vi "Day 6.2 - .vi"(11 "input":string) -> (3 "output":i16)   [LabVIEW 2021]
uses:
  c0392e8e-aec3-4db0-a7c0-dbb49c44d685.vi
  <vilib>/Comparison/Less/Less Functor/Less Functor.lvclass
panel:
  # "mjqjpqmgbljsphdztnvjfqwrcgsmlb: first marker after character 19\nbvwbjplbgvbhsrlpgdmjqwftvncz: first marker after character 23\nnppdvjthqldpwncqszvftbrmjlhg: first marker after character 23\nnznrnfrfntjfmvfwmzdfjlvtqnbhcprsg: first marker after character 29\nzcfzfwzzqfrljwzlrfnpqdbhtmscgvjw: first marker after character 26"
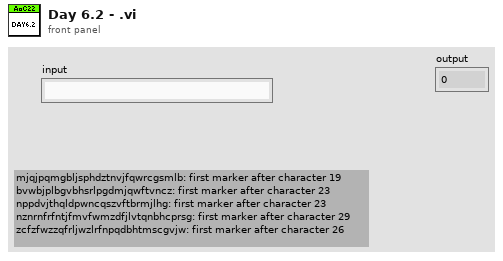
[diagram p1: front panel]
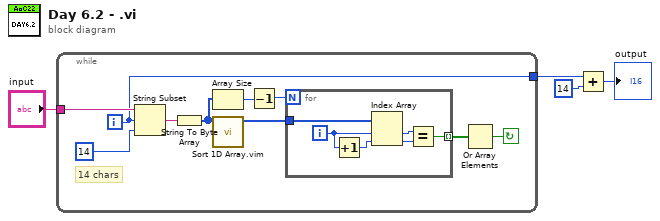
[diagram p0: block diagram]
diagram:
  n1 = while {
    tunnel: "input" -> [w14]
    tunnel: [w11] -> w3
    i -> [w11]
    stop <- w5 continue-if-true
    # "14 chars"
    n2 = String Subset(string=w14, offset (0)=w11, length (rest)=14 ("length (rest)")) -> (substring=w12:string)
    n3 = String To Byte Array(string=w12) -> (unsigned byte array=w9:u8[])
    n4 = Array Size(array=w9) -> (size(s)=w7:i32)
    n5 = call "Sort 1D Array.vim"("unsorted array"=w9) -> ("sorted array"=w10:u8[])  [unwired: 10 in]
    n6 = Decrement(x=w7) -> (x-1=w8:i32)
    n7 = for {
      N: w8 -> [_]
      tunnel: w10 -> [w20]
      tunnel: [w15] -> w6 mode=indexing
      i -> [w18]
      n8 = Increment(x=w18) -> (x+1=w19:i32)
      n9 = Index Array(array=w20, index #1=w18, index #2=w19) -> (element #1=w16:u8, element #2=w17:u8)
      n10 = Equal?(x=w16, y=w17) -> (x = y?=w15:bool)
    }
    n11 = Or Array Elements(Boolean array=w6) -> (logical OR=w5:bool)
  }
  n12 = Add(x=w3, y=14) -> (x+y=→"output":i32)
